vi "RamCtrl_RelTraj_Work.vi"(5 "Track Width FT":dbl, 7 "Max Speed\nFT/SEC":dbl, 8 "Init":bool, 9 "Gyro Continous\n (inc counterclockwise)\nDEG":dbl, 10 "Right Distance FT":dbl, 11 "Left Distance FT":dbl) -> (0 "AtReference":bool, 1 "Right Speed Target":dbl, 2 "Left Speed Target":dbl, 4 "Odometry Pose Meters":T1={"TRANSLATION"={"X"=0.0, "Y"=0.0}, "ROTATION"={"VALUE"=0.0, "COS"=1.0, "SIN"=0.0}} {"ROTATION"."SIN" format="%13.4f"; "ROTATION"."COS" format="%13.4f"; "ROTATION"."VALUE" format="%13.4f"; "TRANSLATION"."Y" format="%14.3f"; "TRANSLATION"."X" format="%14.3f"})   [LabVIEW 2019]
uses:
  <vilib>/Rock Robotics/WPI/ThirdParty/JAS_Junk/TrajLib/Trajectory_Library.lvlib
  RamCtrl_Traj_Globals.vi
  <vilib>/Rock Robotics/WPI/ThirdParty/JAS_Junk/TrajLib/TypeDef/TRANSLATION2D.ctl
  <vilib>/Rock Robotics/WPI/ThirdParty/JAS_Junk/TrajLib/TypeDef/ROTATION2D.ctl
  <vilib>/Rock Robotics/WPI/ThirdParty/JAS_Junk/TrajLib/TypeDef/POSE2D.ctl
panel:
  in  "Add Vision Meas":bool
  in  "visionRobotPose":T1={"TRANSLATION"={"X"=0.0, "Y"=0.0}, "ROTATION"={"VALUE"=0.0, "COS"=1.0, "SIN"=0.0}} {"ROTATION"."SIN" format="%13.4f"; "ROTATION"."COS" format="%13.4f"; "ROTATION"."VALUE" format="%13.4f"; "TRANSLATION"."Y" format="%14.3f"; "TRANSLATION"."X" format="%14.3f"}
  in  "Vision TImeStamp_Seconds":dbl=0.02
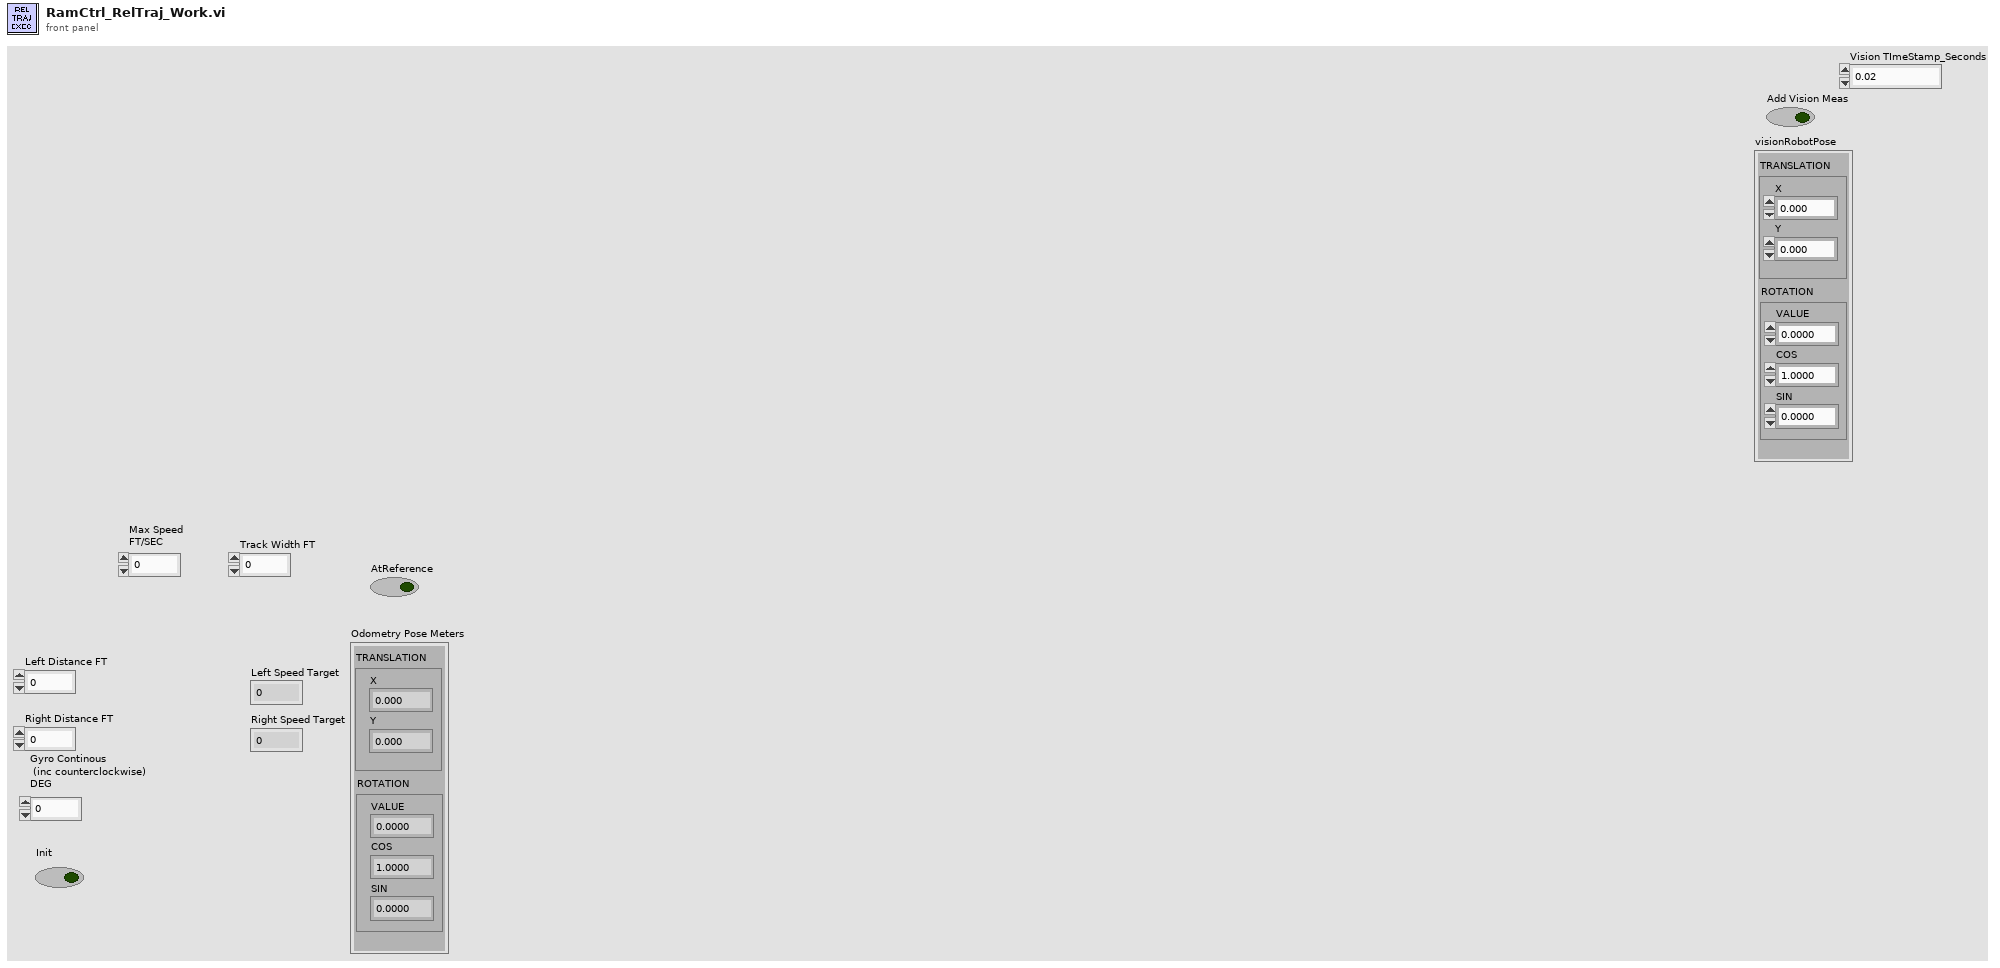
[diagram p1: front panel]
types:
  T1 = typedef "Trajectory_Library.lvlib/POSE2D.ctl" = cluster{"TRANSLATION":T2, "ROTATION":T3}
  T2 = typedef "Trajectory_Library.lvlib/TRANSLATION2D.ctl" = cluster{"X":dbl, "Y":dbl}
  T3 = typedef "Trajectory_Library.lvlib/ROTATION2D.ctl" = cluster{"VALUE":dbl, "COS":dbl, "SIN":dbl}
  T4 = typedef "Trajectory_Library.lvlib/TRAJECTORY.ctl" = cluster{"TotalTImeSecs":dbl, "States":T5[]}
  T5 = typedef "Trajectory_Library.lvlib/TRAJ_STATE.ctl" = cluster{"TimeSeconds":dbl, "Velocity":dbl, "Acceleration":dbl, "POSE":T1, "Curvature":dbl}
  T6 = typedef "Trajectory_Library.lvlib/RAMSETE_EXE_TUNING.ctl" = cluster{"B":dbl, "Zeta":dbl, "X Tolerance M":dbl, "Y Tolerance M":dbl, "Heading Tolerance RAD":dbl, "Track Width M":dbl, "Max Speed M/S":dbl}
  T7 = typedef "Trajectory_Library.lvlib/DIFF_DRIVE_POSE_EST2_CONFIG.ctl" = cluster{"TrackWidth_Meters":dbl, "Odom X std dev M":dbl, "Odom Y std dev M":dbl, "Odom Heading std dev Rad":dbl, "Vision X std dev M":dbl, "Vision Y std dev M":dbl, "Vision Heading std dev Rad":dbl}
  T8 = typedef "Trajectory_Library.lvlib/RAMSETE.ctl" = cluster{"B":dbl, "Zeta":dbl, "poseTolerance":T1, "poseError":T1, "Enabled":bool}
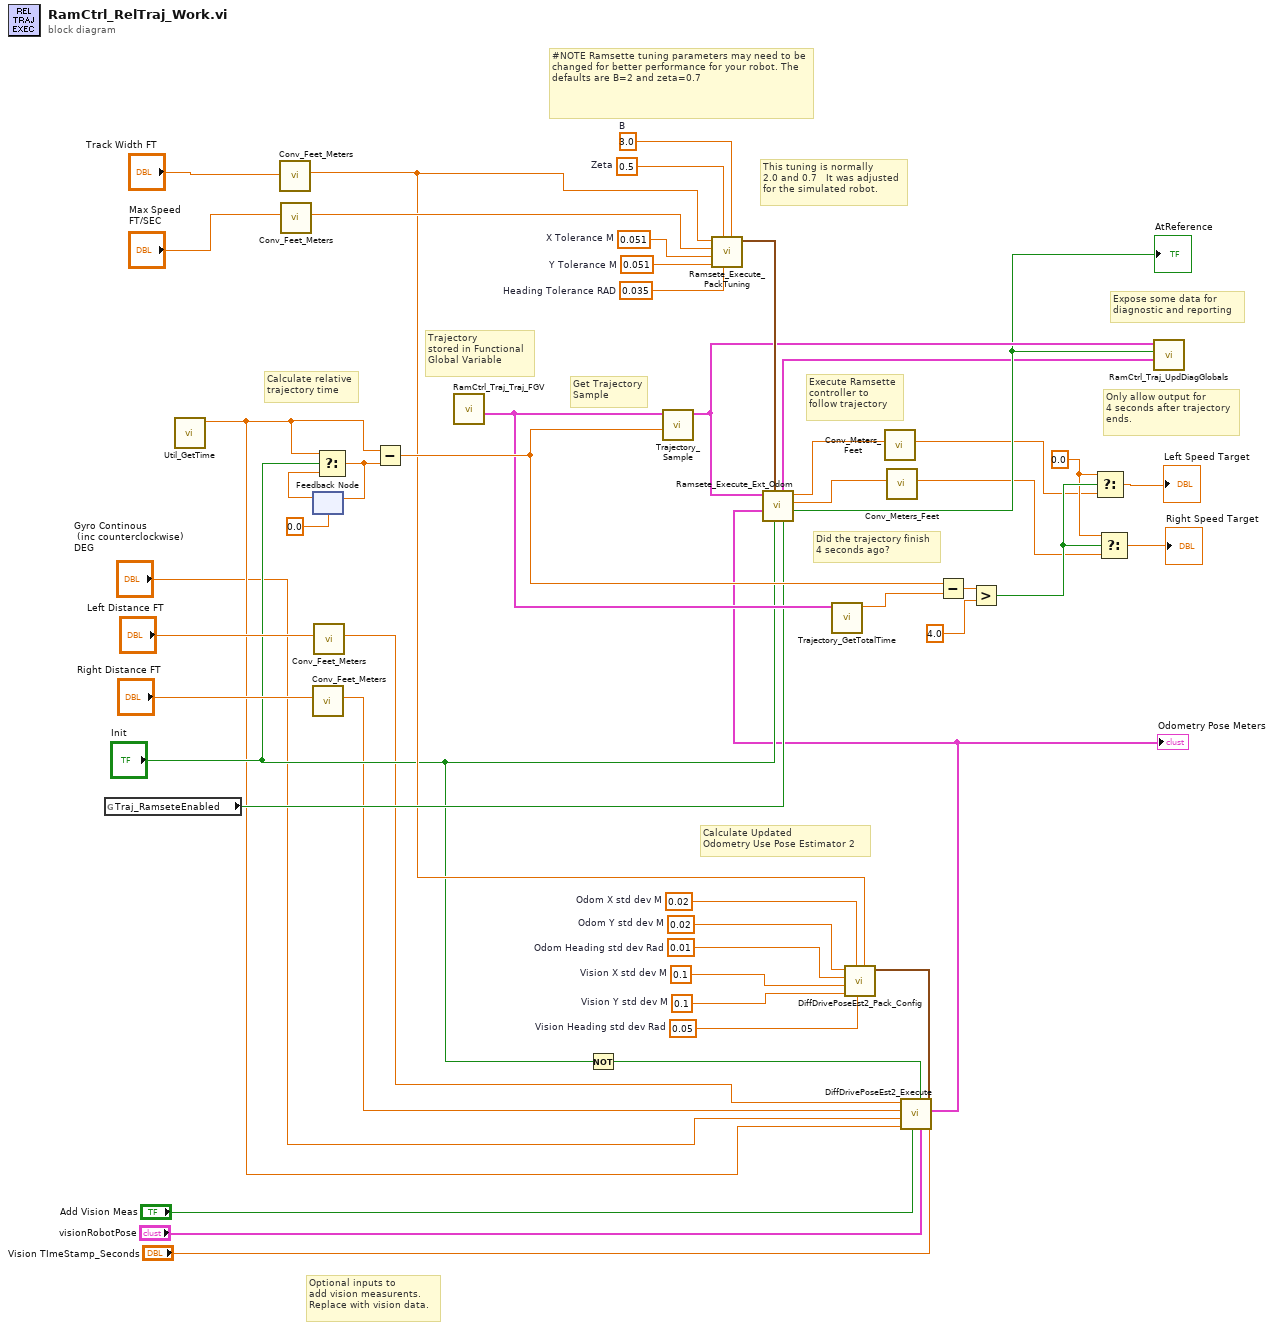
[diagram p0: block diagram]
diagram:
  w12 = 0.02  # Odom Y std dev M
  w13 = 0.01  # Odom Heading std dev Rad
  w14 = 0.1  # Vision X std dev M
  w15 = 0.1  # Vision Y std dev M
  w16 = 0.02  # Odom X std dev M
  w17 = 0.05  # Vision Heading std dev Rad
  w37 = 0.051  # X Tolerance M
  w36 = 0.051  # Y Tolerance M
  w35 = 0.5  # Zeta
  w34 = 0.035  # Heading Tolerance RAD
  w33 = 3.0  # B
  w44 = 0.0 ("t")
  # "Optional inputs to\nadd vision measurents.\nReplace with vision data."
  # "Execute Ramsette\ncontroller to \nfollow trajectory"
  # "Calculate Updated\nOdometry Use Pose Estimator 2"
  # "This tuning is normally\n2.0 and 0.7   It was adjusted\nfor the simulated robot."
  # "Expose some data for\ndiagnostic and reporting"
  # "Did the trajectory finish\n4 seconds ago?"
  # "Get Trajectory\nSample"
  # "Trajectory\nstored in Functional\nGlobal Variable"
  # "Calculate relative\ntrajectory time"
  # "#NOTE Ramsette tuning parameters may need to be changed for better performance for your robot. The defaults are B=2 and zeta=0.7"
  # "Only allow output for\n4 seconds after trajectory\nends."
  n1 = global read "RamCtrl_Traj_Globals.vi" "Traj_RamseteEnabled"() -> (w28:bool)
  n2 = call <vilib>:"Util_GetTime.vi"() -> ("FPGA_Time_Seconds"=w4:dbl)  [unwired: 9 in, 2 out]
  n3 = call <vilib>:"Conv_Feet_Meters.vi"("Feet"="Track Width FT") -> ("Meters"=w8:dbl)  [unwired: 10 in]
  n4 = call <vilib>:"Conv_Feet_Meters.vi"("Feet"="Max Speed\nFT/SEC") -> ("Meters"=w31:dbl)  [unwired: 10 in]
  n5 = feedback #1(0.0 ("TIME")) -> (w40:dbl)
  n6 = call <vilib>:"Conv_Feet_Meters.vi"("Feet"="Right Distance FT") -> ("Meters"=w5:dbl)  [unwired: 10 in]
  n7 = call <vilib>:"Conv_Feet_Meters.vi"("Feet"="Left Distance FT") -> ("Meters"=w2:dbl)  [unwired: 10 in]
  n8 = Select(t=w4, s="Init", f=w40) -> (s? t:f=w41:dbl)
  n9 = feedback-in #1(w41) -> ()
  n10 = Subtract(x=w4, y=w41) -> (x-y=w48:dbl)
  n11 = call "RamCtrl_Traj_Traj_FGV.vi"() -> ("outTRAJECTORY"=w39:T4)  [unwired: 11 in]
  n12 = Not(x="Init") -> (.not. x?=w7:bool)
  n13 = call <vilib>:"Trajectory_Sample.vi"("Time"=w48, "InputTRAJECTORY"=w39) -> ("OutputTRAJ_STATE"=w25:T5)  [unwired: 9 in]
  n14 = call <vilib>:"Ramsete_Execute_PackTuning.vi"("B"=w33, "Heading Tolerance RAD"=w34, "Zeta"=w35, "Y Tolerance M"=w36, "X Tolerance M"=w37, "Max Speed M/S"=w31, "Track Width M"=w8) -> ("RAMSETE_EXE_TUNING"=w32:T6)  [unwired: 4 in]
  n15 = call <vilib>:"Trajectory_GetTotalTime.vi"("TRAJECTORY"=w39) -> ("TotalTime_Sec"=w38:dbl)  [unwired: 10 in]
  n16 = call <vilib>:"DiffDrivePoseEst2_Pack_Config.vi"("TrackWidth_Meters"=w8, "Vision Heading std dev Rad"=w17, "Odom X std dev M"=w16, "Vision Y std dev M"=w15, "Vision X std dev M"=w14, "Odom Heading std dev Rad"=w13, "Odom Y std dev M"=w12) -> ("DiffPoseEst2Config"=w18:T7)  [unwired: 4 in]
  n17 = call <vilib>:"DiffDrivePoseEst2_Execute.vi"("Vision TImeStamp_Seconds"="Vision TImeStamp_Seconds", "DiffPoseEst2Config"=w18, "visionRobotPose"="visionRobotPose", "Game Started"=w7, "Add Vision Meas"="Add Vision Meas", "Pass Through Time"=w4, "Gyro Degrees"="Gyro Continous\n (inc counterclockwise)\nDEG", "RightDistance_M"=w5, "LeftDistance_M"=w2) -> ("Estimated Pose"=w1:T1)  [unwired: 1 in, 1 out]
  "Odometry Pose Meters" <- w1
  n18 = call <vilib>:"Ramsete_Execute_Ext_Odom.vi"("Enabled"=w28, "Reset"="Init", "RAMSETE_EXE_TUNING SI"=w32, "Current Pose SI"=w1, "TRAJ_STATE SI"=w25) -> ("AtReference"=w24:bool, "Right Speed Dmd M/S"=w21:dbl, "Left Speed Dmd M/S"=w22:dbl, "outRAMSETE"=w23:T8)  [unwired: 3 in]
  "AtReference" <- w24
  n19 = call <vilib>:"Conv_Meters_Feet.vi"("Meters"=w22) -> ("Feet"=w20:dbl)  [unwired: 10 in]
  n20 = call <vilib>:"Conv_Meters_Feet.vi"("Meters"=w21) -> ("Feet"=w19:dbl)  [unwired: 10 in]
  n21 = Subtract(x=w48, y=w38) -> (x-y=w47:dbl)
  n22 = Greater?(x=w47, y=4.0) -> (0:w45:bool)
  n23 = Select(t=w44, s=w45, f=w20) -> (s? t:f=→"Left Speed Target":dbl)
  n24 = Select(t=w44, s=w45, f=w19) -> (s? t:f=→"Right Speed Target":dbl)
  n25 = call "RamCtrl_Traj_UpdDiagGlobals.vi"("outRAMSETE (SI)"=w23, "AtReference"=w24, "OutputTRAJ_STATE (SI)"=w25) -> ()  [unwired: 9 in]
